vi "Create Wait Events.vi"(8 "error in (no error)":errorcluster) -> (0 "error out":errorcluster, 3 "Wait User Events":T1)   [LabVIEW 2023, in "Weather Wait Loop.lvlib"]
doc: "Creates the user events used by the wait message loop."
uses:
  Weather Wait Loop.lvlib
  User Events.ctl
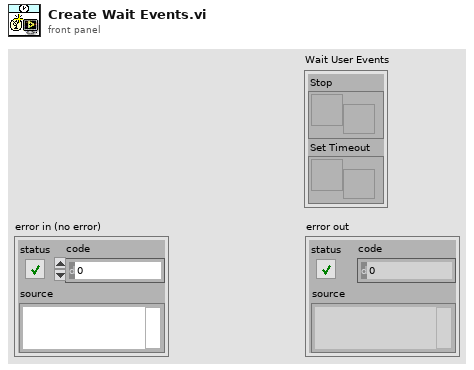
[diagram p1: front panel]
types:
  T1 = typedef "Weather Wait Loop.lvlib/User Events.ctl" = cluster{"Stop":refnum<user-event>, "Set Timeout":refnum<user-event>}
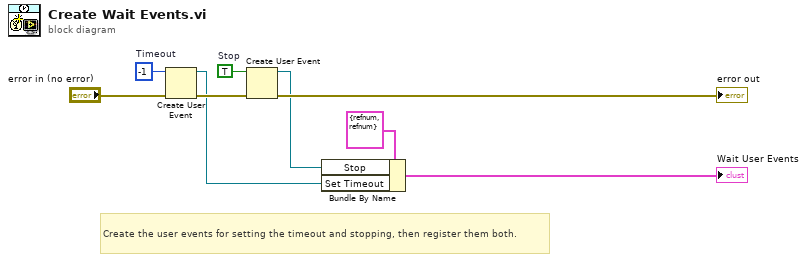
[diagram p0: block diagram]
diagram:
  w7 = TRUE  # Stop
  w8 = -1  # Timeout
  # "Create the user events for setting the timeout and stopping, then register them both."
  n1 = Create User Event(user event datatype=w8, error in="error in (no error)") -> (user event=w3:refnum<user-event>, error out=w9:errorcluster)
  n2 = Create User Event(user event datatype=w7, error in=w9) -> (user event=w4:refnum<user-event>, error out=→"error out":errorcluster)
  n3 = Bundle By Name(cluster=T1 {"Stop"=refnum, "Set Timeout"=refnum} ("Wait User Events"), "Stop"=w4, "Set Timeout"=w3) -> (→"Wait User Events":T1)
